vi "appendXMLImageServer.vi"(8 "error in (no error)":errorcluster, 9 "ImageServer":cluster{"IPAddress":string, "Port":i32}, 10 "Parent Camera Node":refnum<k20>, 11 "DOM document in":refnum<k20>) -> (0 "error out":errorcluster)   [LabVIEW 2013]
uses:
  <resource>/objmgr/DOMUserDefRef.rc
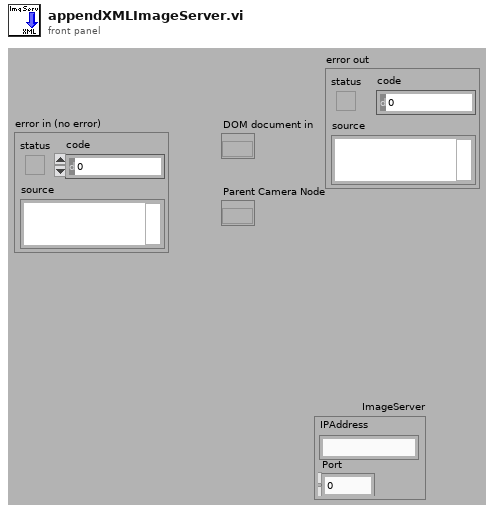
[diagram p1: front panel]
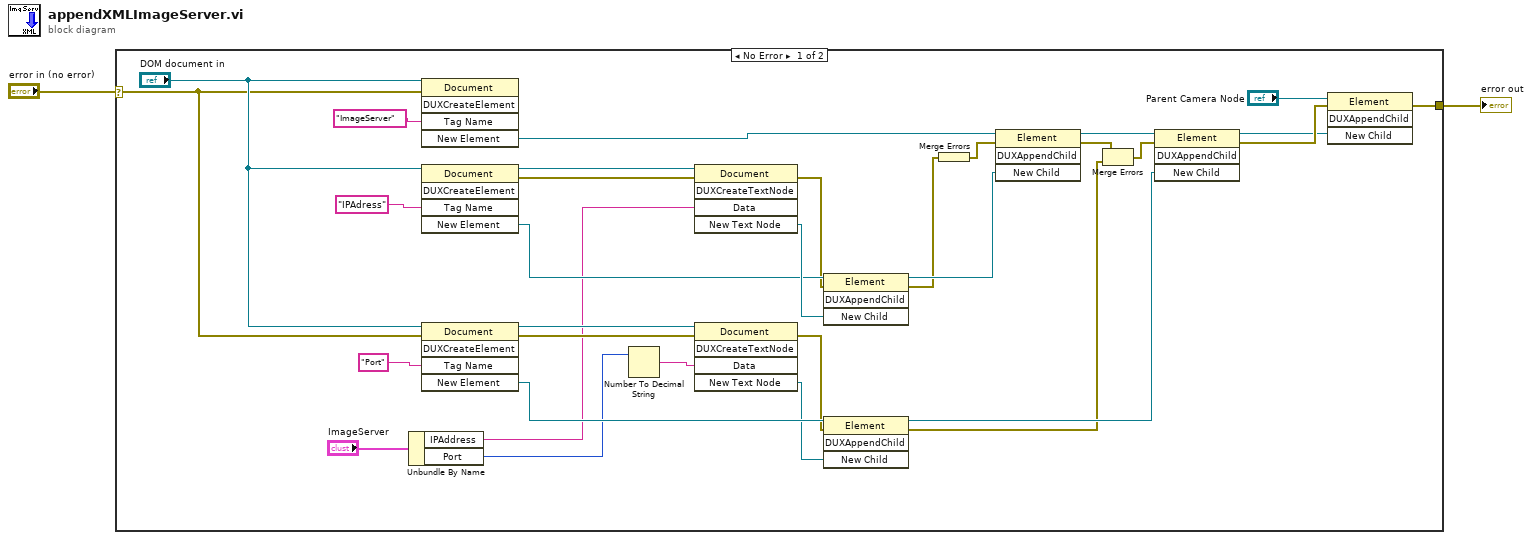
[diagram p0: block diagram]
diagram:
  n1 = case shown="No Error" "error in (no error)" {
    selector: "error in (no error)" -> [w7 w35]
    tunnel: [w10 w35] -> w2
    frame No Error {
      n2 = Unbundle By Name("ImageServer") -> ("IPAddress"=w9:string, "Port"=w8:i32)
      n3 = invoke class="Document" method="DUXCreateElement"(reference="DOM document in", error in=w7, "Tag Name"="ImageServer") -> ("New Element"=w5:refnum<k20>)  [unwired: 2 in, 4 out]
      n4 = invoke class="Document" method="DUXCreateElement"(reference="DOM document in", "Tag Name"="IPAdress") -> (reference out=w32:refnum<k20>, error out=w19:errorcluster, "New Element"=w30:refnum<k20>)  [unwired: 3 in, 2 out]
      n5 = invoke class="Document" method="DUXCreateElement"(reference="DOM document in", error in=w7, "Tag Name"="Port") -> (reference out=w25:refnum<k20>, error out=w18:errorcluster, "New Element"=w27:refnum<k20>)  [unwired: 2 in, 2 out]
      n6 = Number To Decimal String(number=w8) -> (decimal integer string=w20:string)  [unwired: 1 in]
      n7 = invoke class="Document" method="DUXCreateTextNode"(reference=w32, error in=w19, "Data"=w9) -> (error out=w17:errorcluster, "New Text Node"=w31:refnum<k20>)  [unwired: 2 in, 3 out]
      n8 = invoke class="Document" method="DUXCreateTextNode"(reference=w25, error in=w18, "Data"=w20) -> (error out=w16:errorcluster, "New Text Node"=w26:refnum<k20>)  [unwired: 2 in, 3 out]
      n9 = invoke class="Element" method="DUXAppendChild"(reference=w30, error in=w17, "New Child"=w31) -> (reference out=w29:refnum<k20>, error out=w14:errorcluster)  [unwired: 1 in, 2 out]
      n10 = invoke class="Element" method="DUXAppendChild"(reference=w27, error in=w16, "New Child"=w26) -> (reference out=w22:refnum<k20>, error out=w11:errorcluster)  [unwired: 1 in, 2 out]
      n11 = Merge Errors(w14) -> (w15:errorcluster)
      n12 = invoke class="Element" method="DUXAppendChild"(reference=w5, error in=w15, "New Child"=w29) -> (reference out=w23:refnum<k20>, error out=w12:errorcluster)  [unwired: 1 in, 2 out]
      n13 = Merge Errors(w12, w11) -> (w13:errorcluster)
      n14 = invoke class="Element" method="DUXAppendChild"(reference=w23, error in=w13, "New Child"=w22) -> (reference out=w3:refnum<k20>, error out=w4:errorcluster)  [unwired: 1 in, 2 out]
      n15 = invoke class="Element" method="DUXAppendChild"(reference="Parent Camera Node", error in=w4, "New Child"=w3) -> (error out=w10:errorcluster)  [unwired: 1 in, 3 out]
    }
    frame Error {
    }
  }
  "error out" <- w2
